vi "Sub_Online_Plotter.vi"(10 "Experiment":T3) -> (3 "Plotables":T1)   [LabVIEW 2021]
panel:
  out "Plotables":T2
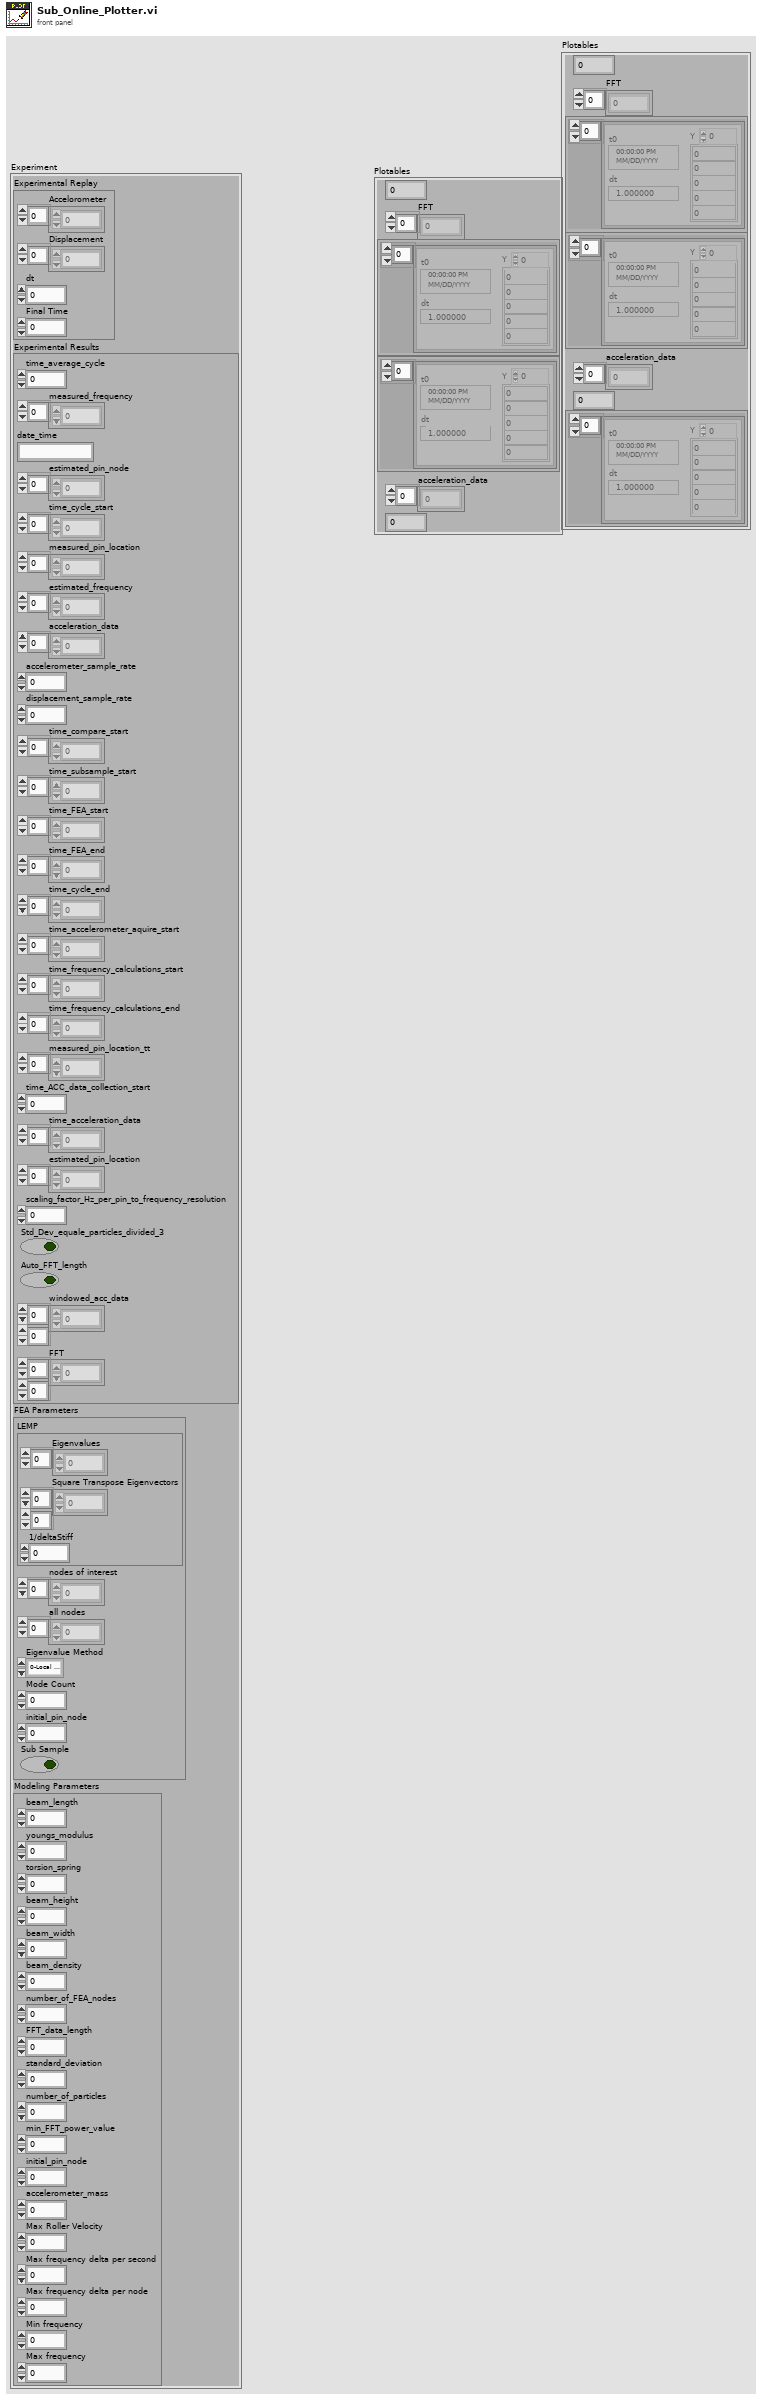
[diagram p1: front panel]
types:
  T1 = cluster{dbl, "FFT":dbl[], "Dynamic Data":dynamicdata, "Dynamic Data":dynamicdata, "acceleration_data":dbl[], dbl, "Dynamic Data":dynamicdata}
  T2 = cluster{dbl, "FFT":dbl[], "Dynamic Data":dynamicdata, "Dynamic Data":dynamicdata, "acceleration_data":dbl[], dbl}
  T3 = cluster{"Experimental Replay":cluster{"Accelorometer":dbl[], "Displacement":dbl[], "dt":dbl, "Final Time":dbl}, "Experimental Results":cluster{"time_average_cycle":dbl, "measured_frequency":dbl[], "date_time":string, "estimated_pin_node":i32[], "time_cycle_start":dbl[], "measured_pin_location":dbl[], "estimated_frequency":dbl[], "acceleration_data":dbl[], "accelerometer_sample_rate":dbl, "displacement_sample_rate":dbl, "time_compare_start":dbl[], "time_subsample_start":dbl[], "time_FEA_start":dbl[], "time_FEA_end":dbl[], "time_cycle_end":dbl[], "time_accelerometer_aquire_start":dbl[], "time_frequency_calculations_start":dbl[], "time_frequency_calculations_end":dbl[], "measured_pin_location_tt":dbl[], "time_ACC_data_collection_start":dbl, "time_acceleration_data":dbl[], "estimated_pin_location":dbl[], "scaling_factor_Hz_per_pin_to_frequency_resolution":dbl, "Std_Dev_equale_particles_divided_3":bool, "Auto_FFT_length":bool, "windowed_acc_data":dbl[][], "FFT":dbl[][]}, "FEA Parameters":cluster{"LEMP":cluster{"Eigenvalues":dbl[], "Square Transpose Eigenvectors":dbl[][], "1/deltaStiff":dbl}, "nodes of interest":i32[], "all nodes":i32[], "Eigenvalue Method":enum16{"0-Local Eigen Modification Procedure", "1-LabVIEW generalized eigenvalues", "2-LabVIEW M^-1K eigenvalues", "3-LabVIEW Cholesky Factorization", "4-Cholesky Factorization CPU SGL", "5-Cholesky Factorization CPU FXP", "6-Cholesky Factorization FPGA SGL", "7-Cholesky Factorization FPGA SGL SCL"}, "Mode Count":i32, "initial_pin_node":i32, "Sub Sample":bool}, "Modeling Parameters":cluster{"beam_length":dbl, "youngs_modulus":dbl, "torsion_spring":dbl, "beam_height":dbl, "beam_width":dbl, "beam_density":dbl, "number_of_FEA_nodes":i32, "FFT_data_length":i32, "standard_deviation":dbl, "number_of_particles":i32, "min_FFT_power_value":dbl, "initial_pin_node":i32, "accelerometer_mass":dbl, "Max Roller Velocity":dbl, "Max frequency delta per second":dbl, "Max frequency delta per node":dbl, "Min frequency":dbl, "Max frequency":dbl}}
  T4 = cluster{dbl, "FFT":dbl[], dynamicdata, dynamicdata, "acceleration_data":dbl[], dbl, dynamicdata}
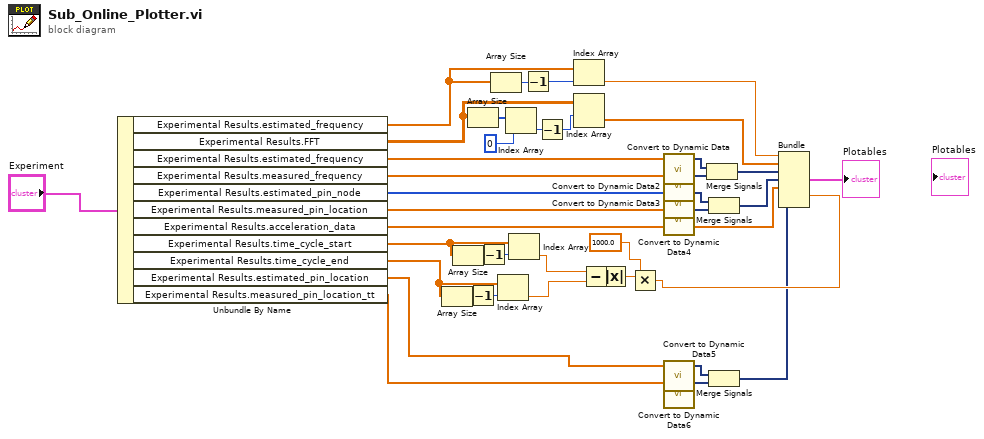
[diagram p0: block diagram]
diagram:
  n1 = Unbundle By Name("Experiment") -> ("Experimental Results.estimated_frequency"=w32:dbl[], "Experimental Results.FFT"=w36:dbl[][], "Experimental Results.estimated_frequency"=w38:dbl[], "Experimental Results.measured_frequency"=w37:dbl[], "Experimental Results.estimated_pin_node"=w39:i32[], "Experimental Results.measured_pin_location"=w40:dbl[], "Experimental Results.acceleration_data"=w10:dbl[], "Experimental Results.time_cycle_start"=w23:dbl[], "Experimental Results.time_cycle_end"=w18:dbl[], "Experimental Results.estimated_pin_location"=w5:dbl[], "Experimental Results.measured_pin_location_tt"=w1:dbl[])
  n2 = Array Size(array=w18) -> (size(s)=w20:i32)
  n3 = Array Size(array=w23) -> (size(s)=w22:i32)
  n4 = Array Size(array=w36) -> (size(s)=w35:i32[])
  n5 = Decrement(x=w20) -> (x-1=w19:i32)
  n6 = Decrement(x=w22) -> (x-1=w21:i32)
  n7 = Array Size(array=w32) -> (size(s)=w31:i32)
  n8 = Index Array(array=w18, index=w19) -> (element=w17:dbl)
  n9 = Index Array(array=w35, index=0) -> (element=w33:i32)
  n10 = Index Array(array=w23, index=w21) -> (element=w16:dbl)
  n11 = Decrement(x=w31) -> (x-1=w30:i32)
  n12 = Decrement(x=w33) -> (x-1=w11:i32)
  n13 = Index Array(array=w32, index=w30) -> (element=w13:dbl)
  n14 = Index Array(array=w36, index (row)=w11) -> (element=w12:dbl[])  [unwired: 1 in]
  n15 = Subtract(x=w16, y=w17) -> (x-y=w29:dbl)
  n16 = Absolute Value(x=w29) -> (abs(x)=w28:dbl)
  n17 = Multiply(x=w28, y=1000.0) -> (x*y=w9:dbl)
  n18 = call "Convert to Dynamic Data"("Array"=w38) -> ("Dynamic Data Type"=w27:dynamicdata)  [unwired: 3 in]
  n19 = call "Convert to Dynamic Data2"("Array"=w37) -> ("Dynamic Data Type"=w26:dynamicdata)  [unwired: 3 in]
  n20 = call "Convert to Dynamic Data3"("Array"=w39) -> ("Dynamic Data Type"=w25:dynamicdata)  [unwired: 3 in]
  n21 = call "Convert to Dynamic Data4"("Array"=w40) -> ("Dynamic Data Type"=w24:dynamicdata)  [unwired: 3 in]
  n22 = call "Convert to Dynamic Data5"("Array"=w5) -> ("Dynamic Data Type"=w7:dynamicdata)  [unwired: 3 in]
  n23 = call "Convert to Dynamic Data6"("Array"=w1) -> ("Dynamic Data Type"=w6:dynamicdata)  [unwired: 3 in]
  n24 = Merge Signals(w27, w26) -> (w15:dynamicdata)
  n25 = Merge Signals(w25, w24) -> (w14:dynamicdata)
  n26 = Merge Signals(w7, w6) -> (w3:dynamicdata)
  n27 = Bundle(w13, "FFT"=w12, w15, w14, "acceleration_data"=w10, w9, w3) -> (→"Plotables":T4)  [unwired: 1 in]
